vi "encoder2_test_v3.vi"() -> ()   [LabVIEW 2014]
uses:
  <vilib>/rvi/FXPMathLib/FxpSinAndCos/subVIs/nifxpmath_SinAndCos_SimConfig.ctl
  <vilib>/rvi/Emulation/niFpgaGetClockAttributes.vi
  <vilib>/rvi/Emulation/niFpgaSctlEmulationGetInTimedLoop.vi
  <vilib>/rvi/Emulation/niFpgaEmulationReportErrorSimple.vi
  <vilib>/rvi/eio/common/nirviEmuTemplateMethod_errors.vi
  <vilib>/rvi/Emulation/niFpgaProcessEmulError.vi
  <vilib>/rvi/Emulation/niFpgaCriticalErrorInLSC.vi
  <vilib>/rvi/interface/RandomDataEmulation/nirviRandomDataMultiElementFPGAFIFO.vi
  <instcachedir>/0/nirviRandomDataMultiElementFPGAFIFO_AD0CFC12EF974623A9C2E4184BC062B2.lvgen/nirviRandomDataMultiElementFPGAFIFO_AD0CFC12EF974623A9C2E4184BC062B2_028.vi
  <vilib>/rvi/interface/RandomDataEmulation/niFpgaRandomDataHandleErrors.vi
  <vilib>/rvi/FXPMathLib/FxpSinAndCos/simVIs/DllFxpSinAndCosTemp_sub.vi
  <vilib>/eio/EIONode/EIONode.xnode
  <vilib>/rvi/FXPMathLib/FxpMul/XNode/nifxpmath_Multiplier.xnode
  <vilib>/rvi/DataTransferAndStorage/Container/XNode/niFpgaContainer.xnode
  <vilib>/rvi/interface/RandomDataEmulation/nirviRandomDataFpgaMultiElementTemplate.vi
  <vilib>/rvi/FXPMathLib/FxpSinAndCos/XNode/nifxpmath_SinAndCos.xnode
  <vilib>/rvi/FXPMathLib/FxpSub/XNode/nifxpmath_Sub.xnode
  <vilib>/rvi/FXPMathLib/sim/FxpSim.dll
panel:
  in  "Tc_Mavg_mot (uSec)":i32 caption="D_d_M_avg_Tc (uSec)"
  out "omega_mot (M_avg)":fxp<+/-,40,19>
  out "D_d_mot (M_avg)":fxp<+/-,40,19>
  out "omega_mag 2":fxp<+/-,36,13>
  out "D_d_mag 2":fxp<+/-,36,16>
  in  "Tc_Mavg_mag  (uSec)":i32 caption="D_d_M_avg_Tc (uSec)"
  out "D_d_mag (M_avg)":fxp<+/-,40,19>
  out "omega_mag (M_avg)":fxp<+/-,40,19>
  in  "Velocity Est. (mag)":i16(ring) items=["T method", "Mavg method"]
  out "rad (NrTheta)":fxp<+/-,40,20>
  out "D (mm)":fxp<+/-,32,7>
  out "Dr_ramp2":fxp<+/-,64,21>
  out "Ts (s)":fxp<+/-,32,6>
  in  "Dr_ramp (mm)":fxp<+/-,33,7>
  out "Dr_ramp":fxp<+/-,64,21>
  in  "Vr (mm/s)":fxp<+/-,33,7>
  out "omega (rad/s)":fxp<+/-,36,13>
  in  "Encoder":i16(ring) items=["Motor", "Magnetic"]
  in  "Dr_step":fxp<+/-,33,7>
  out "Dr":fxp<+/-,33,10>
  in  "Command type":i16(ring) items=["Step", "Sine", "Ramp", "Ramp2"]
  out "Fmr_P":fxp<+/-,30,15>
  in  "Kp":fxp<+/-,27,14>
  out "D_error":fxp<+/-,36,11>
  out "Dr_sin_d":fxp<+/-,51,12>
  out "Sin omega":fxp<+,20,4>
  out "Dr_sin":fxp<+/-,33,10>
  in  "Sin Mag.":fxp<+/-,32,7>
  in  "Sine frequency (Hz)":fxp<+,16,5>=2.0
  out "Time now (s)":fxp<+,52,14>
  out "va":fxp<+/-,36,7>
  out "vb":fxp<+/-,37,8>
  out "vd_F":fxp<+/-,20,5>
  out "vq_F":fxp<+/-,20,5> format="%.57g"
  in  "Stop Motor":bool
  in  "Ini coe.":bool
  out "D_d_mag":fxp<+/-,36,13>
  out "omega_mag":fxp<+/-,36,13>
  out "D_mag":fxp<+/-,32,7>
  in  "Mag. factor":fxp<+/-,20,2>
  out "mt_mag.":u32
  out "D_d_mot":fxp<+/-,36,13>
  in  "Belt_screw":fxp<+/-,7,7>
  in  "Belt_motor":fxp<+/-,6,6>
  out "D_mot":fxp<+/-,32,7>
  out "rad_mag.":fxp<+/-,40,20>
  out "rad_mot":fxp<+/-,40,20>
  out "mt":u32
  out "omega_mot":fxp<+/-,36,13>
  in  "mt0":u32
  out "Mag. Encoder Position":i32
  in  "Encoder Reset":bool
  out "Encoder Position":i32
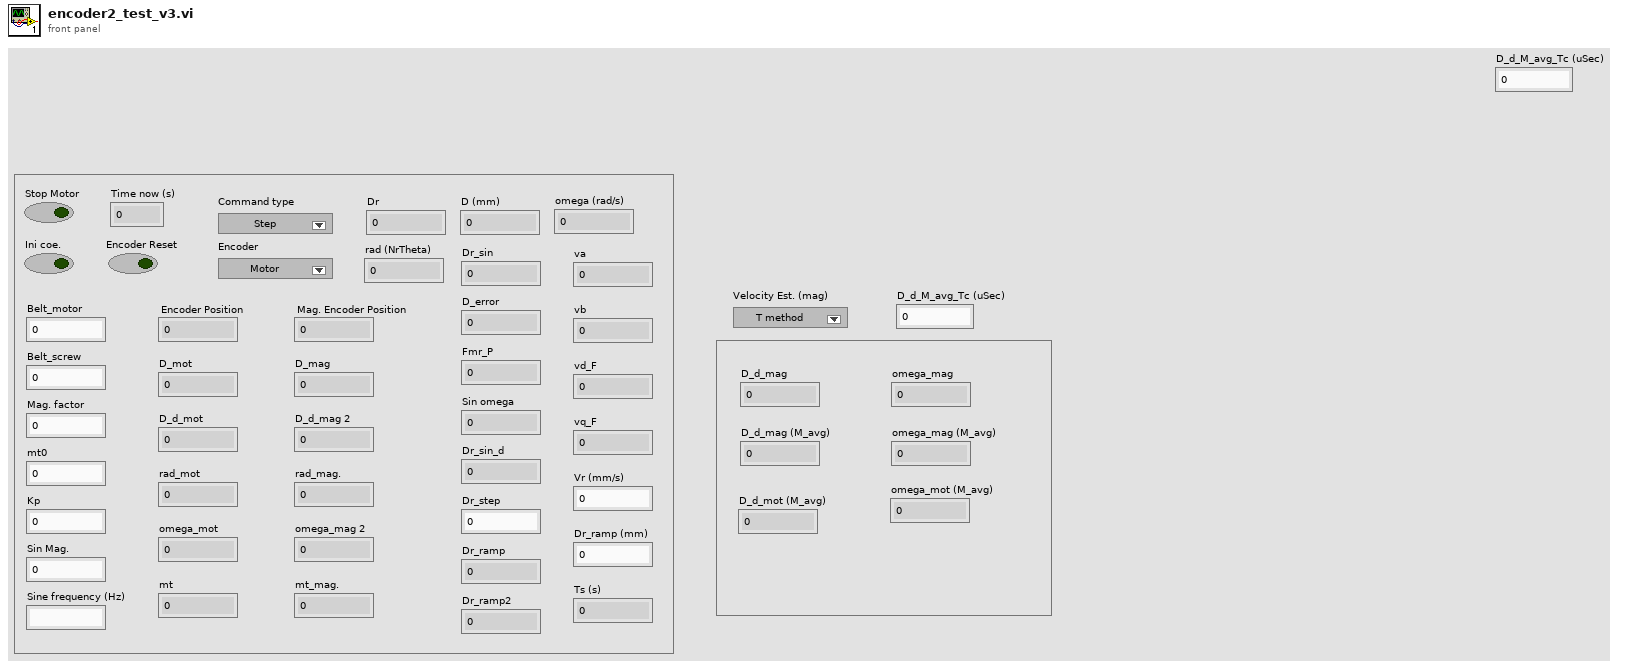
[diagram p1: front panel]
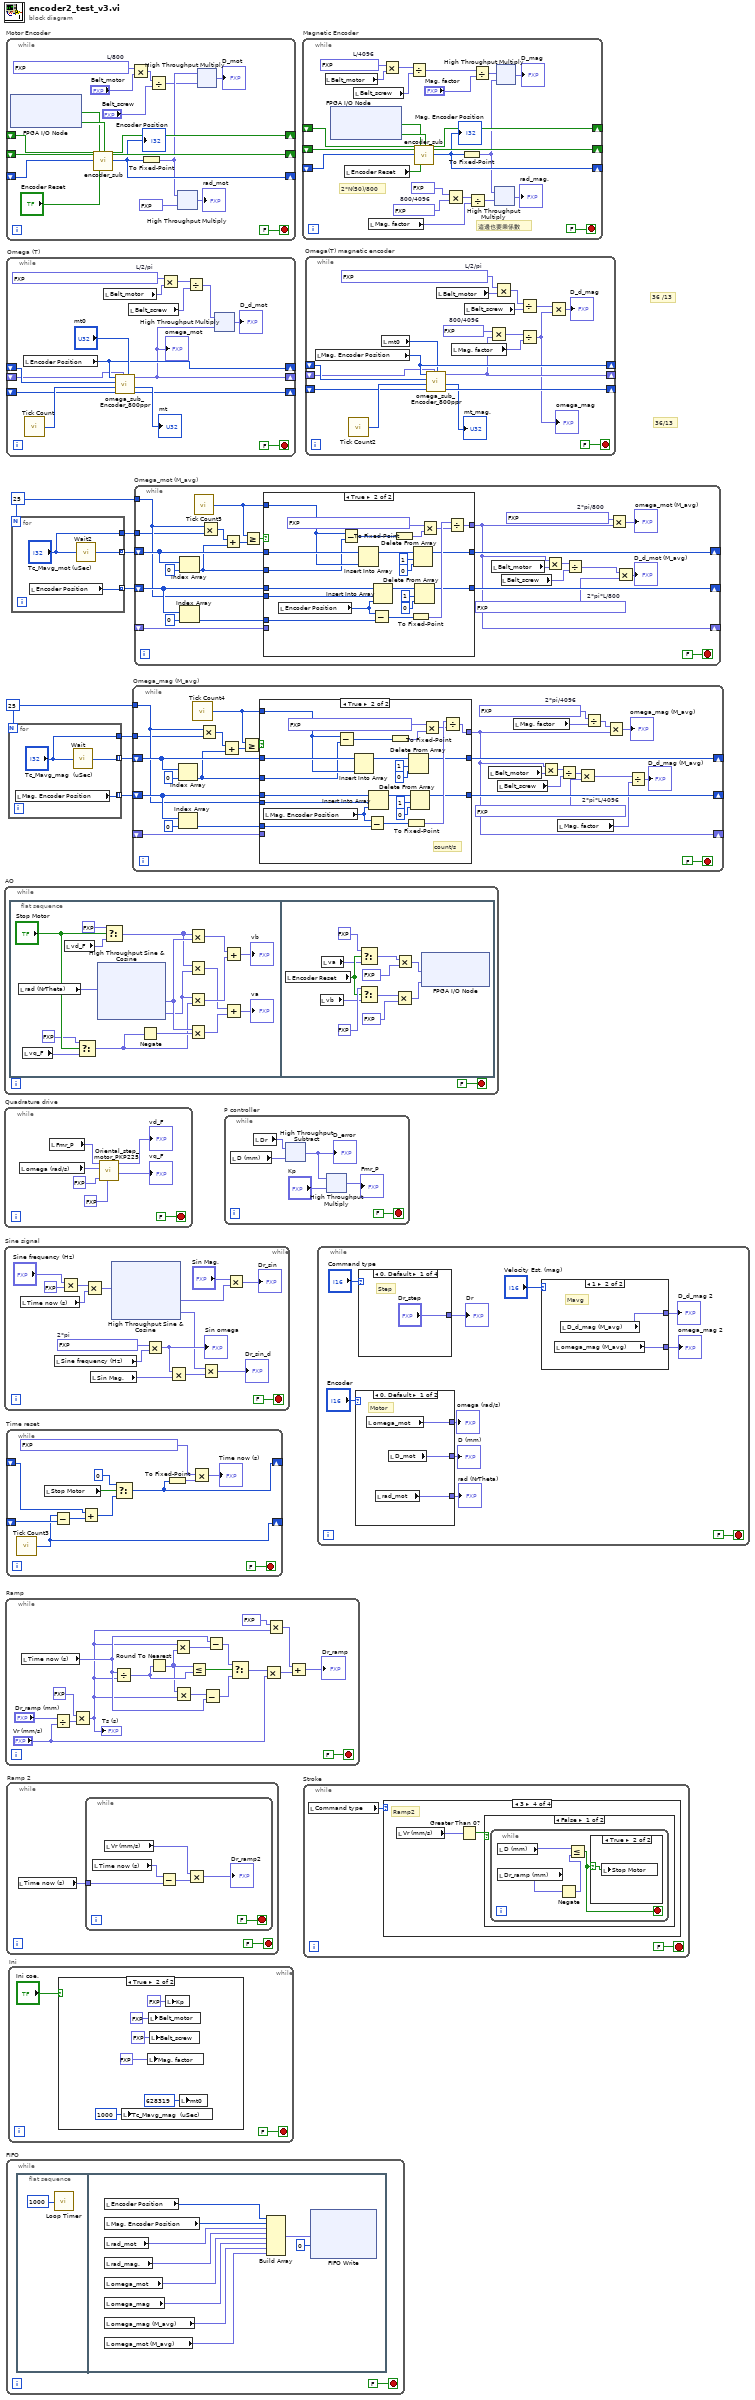
[diagram p0: block diagram]
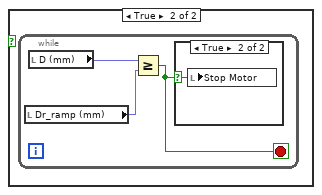
[diagram p8: hidden frame]
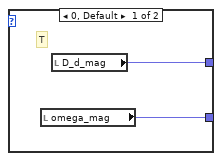
[diagram p10: hidden frame]
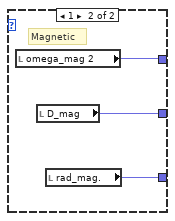
[diagram p11: hidden frame]
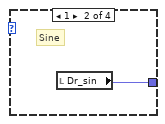
[diagram p12: hidden frame]
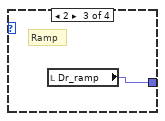
[diagram p13: hidden frame]
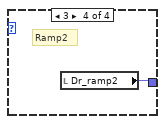
[diagram p14: hidden frame]
diagram:
  w4 = 25
  w8 = 25
  # "36/13"
  # "36 /13"
  n1 = while "AO" {
    stop <- FALSE stop-if-true
    n2 = flat-sequence {
      frame #0 {
        n3 = local read "rad (NrTheta)"() -> (w26:fxp<+/-,40,20>)
        n4 = local read "vq_F"() -> (w22:fxp<+/-,20,5>)
        n5 = local read "vd_F"() -> (w21:fxp<+/-,20,5>)
        n6 = Select(t=fxp<+,1,1> 0.0, s="Stop Motor", f=w22) -> (s? t:f=w12:fxp<+/-,20,5>)
        n7 = xnode "High Throughput Sine & Cosine"("x (pi)"=w26) -> ("sin(x)"=w16:fxp<+/-,16,2>, "cos(x)"=w14:fxp<+/-,16,2>)
        n8 = Select(t=fxp<+,1,1> 0.0, s="Stop Motor", f=w21) -> (s? t:f=w15:fxp<+/-,20,5>)
        n9 = Negate(x=w12) -> (-x=w13:fxp<+/-,21,6>)
        n10 = Multiply(x=w15, y=w16) -> (x*y=w20:fxp<+/-,36,7>)
        n11 = Multiply(x=w15, y=w14) -> (x*y=w18:fxp<+/-,36,7>)
        n12 = Multiply(x=w14, y=w12) -> (x*y=w19:fxp<+/-,36,7>)
        n13 = Multiply(x=w16, y=w13) -> (x*y=w17:fxp<+/-,35,6>)
        n14 = Add(x=w20, y=w19) -> (x+y=→"vb":fxp<+/-,37,8>)
        n15 = Add(x=w18, y=w17) -> (x+y=→"va":fxp<+/-,36,7>)
      }
      frame #1 {
        n16 = local read "Encoder Reset"() -> (w61:bool)
        n17 = local read "vb"() -> (w60:fxp<+/-,37,8>)
        n18 = local read "va"() -> (w59:fxp<+/-,36,7>)
        n19 = Select(t=fxp<+/-,20,5> 3.0 ("y"), s=w61, f=w59) -> (s? t:f=w64:fxp<+/-,36,7>)
        n20 = Select(t=fxp<+/-,20,5> 0.0 ("y"), s=w61, f=w60) -> (s? t:f=w65:fxp<+/-,37,8>)
        n21 = Multiply(x=w65, y=fxp<+/-,20,5> -0.5) -> (x*y=w57:fxp<+/-,55,11>)
        n22 = Multiply(x=w64, y=fxp<+/-,20,5> -0.5) -> (x*y=w58:fxp<+/-,55,11>)
        n23 = xnode "FPGA I/O Node"("Mod8/AO0"=w58, "Mod8/AO1"=w57) -> ()  [unwired: 2 in, 2 out]
      }
    }
  }
  n24 = while "Quadrature drive" {
    stop <- FALSE stop-if-true
    n25 = local read "omega (rad/s)"() -> (w68:fxp<+/-,36,13>)
    n26 = local read "Fmr_P"() -> (w70:fxp<+/-,30,15>)
    n27 = call "Oriental_step_motor_PKP225.vi"("F_Threshold"=fxp<+,12,12> 10.0, "dFmr"=fxp<+,1,1> 0.0 ("t"), "omega"=w68, "Fmr"=w70) -> ("vq_F"=→"vq_F":fxp<+/-,20,5>, "vd_F"=→"vd_F":fxp<+/-,20,5>)  [unwired: 6 in]
  }
  n28 = while "Sine signal" {
    stop <- FALSE stop-if-true
    w84 = fxp<+,20,3> 6.2831878662109375  # 2*pi
    n29 = local read "Time now (s)"() -> (w89:fxp<+,52,14>)
    n30 = local read "Sine frequency (Hz)"() -> (w83:fxp<+,16,5>)
    n31 = Multiply(x="Sine frequency (Hz)", y=fxp<+,1,2> 2.0 ("x")) -> (x*y=w90:fxp<+,16,6>)
    n32 = Multiply(x=w90, y=w89) -> (x*y=w88:fxp<+,64,20>)
    n33 = local read "Sin Mag."() -> (w82:fxp<+/-,32,7>)
    n34 = xnode "High Throughput Sine & Cosine"("x (pi)"=w88) -> ("sin(x)"=w86:fxp<+/-,16,2>, "cos(x)"=w79:fxp<+/-,16,2>)
    n35 = Multiply(x=w84, y=w83) -> (x*y=w81:fxp<+,36,8>)
    "Sin omega" <- w81
    n36 = Multiply(x=w81, y=w82) -> (x*y=w80:fxp<+/-,64,15>)
    n37 = Multiply(x=w79, y=w80) -> (x*y=→"Dr_sin_d":fxp<+/-,64,17>)
    n38 = Multiply(x="Sin Mag.", y=w86) -> (x*y=→"Dr_sin":fxp<+/-,48,9>)
  }
  n39 = while "Ramp" {
    stop <- FALSE stop-if-true
    n40 = local read "Time now (s)"() -> (w134:fxp<+,52,14>)
    n41 = Divide(x="Dr_ramp (mm)", y="Vr (mm/s)") -> (x/y=w123:fxp<+/-,64,34>)
    n42 = Multiply(x=fxp<+/-,3,3> 2.0, y=w123) -> (x*y=w121:fxp<+/-,64,37>)
    "Ts (s)" <- w121
    n43 = Divide(x=w134, y=w121) -> (x/y=w138:fxp<+/-,64,42>)
    n44 = Round To Nearest(number=w138) -> (nearest integer value=w137:fxp<+/-,43,43>)
    n45 = Multiply(x=w121, y=w137) -> (x*y=w136:fxp<+/-,64,79>)
    n46 = Multiply(x=w137, y=w121) -> (x*y=w135:fxp<+/-,64,79>)
    n47 = Less Or Equal?(x=w137, y=w138) -> (x <= y?=w133:bool)
    n48 = Subtract(x=w135, y=w134) -> (x-y=w131:fxp<+/-,64,80>)
    n49 = Subtract(x=w134, y=w136) -> (x-y=w132:fxp<+/-,64,80>)
    n50 = Select(t=w132, s=w133, f=w131) -> (s? t:f=w130:fxp<+/-,64,80>)
    n51 = Multiply(x=w130, y="Vr (mm/s)") -> (x*y=w127:fxp<+/-,64,87>)
    n52 = Multiply(x=fxp<+/-,2,1> -0.5, y=w121) -> (x*y=w126:fxp<+/-,64,38>)
    n53 = Add(x=w126, y=w127) -> (x+y=→"Dr_ramp":fxp<+/-,64,88>)
  }
  n54 = while "Motor Encoder" {
    shift-right: [w155] -> _
    shift-left: _ -> [w156]
    shift-right: [w154] -> _
    shift-left: _ -> [w157]
    shift-right: [w153] -> _
    shift-left: _ -> [w158]
    stop <- FALSE stop-if-true
    w144 = fxp<+/-,20,-5> 0.002499997615814209  # L/800
    n55 = xnode "FPGA I/O Node"() -> ("Mod7/DIO0"=w140:bool, "Mod7/DIO1"=w141:bool)  [unwired: 2 in, 2 out]
    n56 = call "encoder_sub.vi"("A_pre"=w156, "B_pre"=w157, "Encoder Position_pre"=w158, "A input"=w140, "Encoder Position Reset"="Encoder Reset", "B input"=w141) -> ("A"=w155:bool, "B"=w154:bool, "Encoder Position (Counts)"=w153:i32)  [unwired: 19 in]
    "Encoder Position" <- w153
    n57 = Multiply(x=w144, y="Belt_motor") -> (x*y=w146:fxp<+/-,26,1>)
    n58 = To Fixed-Point(number=w153) -> (fixed-point=w148:fxp<+/-,32,32>)  [unwired: 1 in]
    n59 = Divide(x=w146, y="Belt_screw") -> (x/y=w145:fxp<+/-,33,1>)
    n60 = xnode ("High Throughput Multiply")("x"=w148, "y"=fxp<+/-,16,1> 0.125) -> ("x*y"=→"rad_mot":fxp<+/-,48,33>)
    n61 = xnode ("High Throughput Multiply")("x"=w148, "y"=w145) -> ("x*y"=→"D_mot":fxp<+/-,64,33>)
  }
  n62 = while "Time reset" {
    shift-right: [w162] -> _
    shift-left: _ -> [w167]
    shift-right: [w165] -> _
    shift-left: _ -> [w166]
    stop <- FALSE stop-if-true
    n63 = call "Tick Count3"() -> ("Tick Count(uSec)"=w165:u32)
    n64 = local read "Stop Motor"() -> (w170:bool)
    n65 = Subtract(x=w165, y=w166) -> (x-y=w169:u32)
    n66 = Add(x=w167, y=w169) -> (x+y=w168:u32)
    n67 = Select(t=u32 0, s=w170, f=w168) -> (s? t:f=w162:u32)
    n68 = To Fixed-Point(number=w162) -> (fixed-point=w164:fxp<+,32,32>)  [unwired: 1 in]
    n69 = Multiply(x=fxp<+,20,-18> 1.0000003385357559e-06, y=w164) -> (x*y=→"Time now (s)":fxp<+,52,14>)
  }
  n70 = while "FIFO" {
    stop <- FALSE stop-if-true
    n71 = flat-sequence {
      frame #0 {
        n72 = call "Loop Timer"("Count(uSec)"=u32 1000) -> ()  [unwired: 1 out]
      }
      frame #1 {
        n73 = local read "Encoder Position"() -> (w182:i32)
        n74 = local read "Mag. Encoder Position"() -> (w181:i32)
        n75 = local read "rad_mot"() -> (w180:fxp<+/-,40,20>)
        n76 = local read "rad_mag."() -> (w179:fxp<+/-,40,20>)
        n77 = local read "omega_mot"() -> (w178:fxp<+/-,36,13>)
        n78 = local read "omega_mag"() -> (w177:fxp<+/-,36,13>)
        n79 = local read "omega_mag (M_avg)"() -> (w176:fxp<+/-,40,19>)
        n80 = local read "omega_mot (M_avg)"() -> (w173:fxp<+/-,40,19>)
        n81 = Build Array(w182, w181, w180, w179, w178, w177, w176, w173) -> (w174:fxp<+/-,55,32>[])
        n82 = xnode ("FIFO Write")("Element"=w174, "Timeout"=0) -> ()  [unwired: 1 in, 2 out]
      }
    }
  }
  n83 = while "Omega (T)" {
    shift-right: [w196] -> _
    shift-left: _ -> [w197]
    shift-right: [w185] -> _
    shift-left: _ -> [w193]
    shift-right: [w194] -> _
    shift-left: _ -> [w191]
    stop <- FALSE stop-if-true
    w190 = fxp<+/-,32,0> 0.3183098859153688  # L/2/pi
    n84 = local read "Encoder Position"() -> (w196:i32)
    n85 = call "Tick Count"() -> ("Tick Count(Ticks)"=w192:u32)
    n86 = local read "Belt_motor"() -> (w189:fxp<+/-,6,6>)
    n87 = call "omega_sub_Encoder_800ppr.vi"("mt0"="mt0", "omega_pre"=w193, "ticks_m_pre"=w191, "ticks"=w192, "count_pre"=w197, "count"=w196) -> ("ticks_m"=w194:u32, "mt"=→"mt":u32, "omega"=w185:fxp<+/-,36,13>)  [unwired: 3 in]
    "omega_mot" <- w185
    n88 = local read "Belt_screw"() -> (w187:fxp<+/-,7,7>)
    n89 = Multiply(x=w190, y=w189) -> (x*y=w188:fxp<+/-,38,6>)
    n90 = Divide(x=w188, y=w187) -> (x/y=w186:fxp<+/-,45,6>)
    n91 = xnode ("High Throughput Multiply")("x"=w186, "y"=w185) -> ("x*y"=→"D_d_mot":fxp<+/-,64,19>)
  }
  n92 = while "Ramp 2" {
    stop <- FALSE stop-if-true
    n93 = local read "Time now (s)"() -> (w200:fxp<+,52,14>)
    n94 = while {
      tunnel: w200 -> [w205]
      stop <- FALSE stop-if-true
      n95 = local read "Time now (s)"() -> (w206:fxp<+,52,14>)
      n96 = local read "Vr (mm/s)"() -> (w203:fxp<+/-,33,7>)
      n97 = Subtract(x=w206, y=w205) -> (x-y=w204:fxp<+/-,53,15>)
      n98 = Multiply(x=w203, y=w204) -> (x*y=→"Dr_ramp2":fxp<+/-,64,21>)
    }
  }
  n99 = for {
    N: w8 -> [_]
    tunnel: ["Tc_Mavg_mag  (uSec)"] -> w5
    tunnel: [w208] -> w7 mode=indexing
    tunnel: [w207] -> w6 mode=indexing
    n100 = local read "Mag. Encoder Position"() -> (w207:i32)
    n101 = call "Wait"("Count(uSec)"="Tc_Mavg_mag  (uSec)") -> ("Tick Count(uSec)"=w208:u32)
  }
  n102 = while "Ini" {
    stop <- FALSE stop-if-true
    n103 = case shown="True" "Ini coe." {
      frame False {
      }
      frame True {
        n104 = local write "Tc_Mavg_mag  (uSec)"(u32 1000 ("D_d_M_avg_Tc (uSec)")) -> ()
        n105 = local write "Mag. factor"(fxp<+/-,20,2> 1.0 ("Coorection factor")) -> ()
        n106 = local write "Belt_motor"(fxp<+/-,6,6> 14.0 ("Belt_motor")) -> ()
        n107 = local write "Belt_screw"(fxp<+/-,7,7> 36.0 ("Belt_screw")) -> ()
        n108 = local write "Kp"(fxp<+/-,27,14> 50.0 ("Kp")) -> ()
        n109 = local write "mt0"(u32 628319 ("mt0")) -> ()
      }
    }
  }
  n110 = for {
    N: w4 -> [_]
    tunnel: ["Tc_Mavg_mot (uSec)"] -> w2
    tunnel: [w219] -> w3 mode=indexing
    tunnel: [w218] -> w1 mode=indexing
    n111 = local read "Encoder Position"() -> (w218:i32)
    n112 = call "Wait2"("Count(uSec)"="Tc_Mavg_mot (uSec)") -> ("Tick Count(uSec)"=w219:u32)
  }
  n113 = while "Omega_mag (M_avg)" {
    tunnel: w8 -> [w242]
    shift-right: [w235] -> _
    shift-left: w7 -> [w246]
    shift-right: [w221] -> _
    shift-left: _ -> [w237]
    shift-right: [w236] -> _
    shift-left: w6 -> [w245]
    tunnel: w5 -> [w239]
    stop <- FALSE stop-if-true
    w226 = fxp<+/-,27,3> 0.0015339851379394531  # 2*pi/4096
    w229 = fxp<+/-,32,0> 0.003067961661145091  # 2*pi*L/4096
    n114 = Index Array(array=w246, index=0) -> (element=w240:u32)
    n115 = Index Array(array=w245, index=0) -> (element=w241:i32)
    n116 = call "Tick Count4"() -> ("Tick Count(uSec)"=w243:u32)
    n117 = Multiply(x=w242, y=w239) -> (x*y=w247:i32)
    n118 = Add(x=w247, y=w240) -> (x+y=w244:u32)
    n119 = Greater Or Equal?(x=w243, y=w244) -> (x >= y?=w238:bool)
    n120 = case shown="True" w238 {
      tunnel: w246 -> [w252 w269]
      tunnel: w245 -> [w251 w268]
      tunnel: w243 -> [_ w264]
      tunnel: w242 -> [_ w267]
      tunnel: w241 -> [_ w265]
      tunnel: w240 -> [_ w263]
      tunnel: w237 -> [w250 _]
      tunnel: [w251 w259] -> w236
      tunnel: [w252 w258] -> w235
      tunnel: [w250 w257] -> w221
      frame False {
      }
      frame True {
        # "count/s"
        n121 = local read "Mag. Encoder Position"() -> (w266:i32)
        n122 = Subtract(x=w264, y=w263) -> (x-y=w261:u32)
        n123 = Insert Into Array(array=w269, new element=w264) -> (w270:u32[])  [unwired: 1 in]
        n124 = Subtract(x=w266, y=w265) -> (x-y=w256:i32)
        n125 = Insert Into Array(array=w268, index=w267, new element=w266) -> (w271:i32[])
        n126 = To Fixed-Point(number=w261) -> (fixed-point=w253:fxp<+,32,32>)  [unwired: 1 in]
        n127 = To Fixed-Point(number=w256) -> (fixed-point=w260:fxp<+/-,32,32>)  [unwired: 1 in]
        n128 = Delete From Array(array=w270, length=1, index=0) -> (array with subset deleted=w258:u32[])  [unwired: 1 out]
        n129 = Delete From Array(array=w271, length=1, index=0) -> (array with subset deleted=w259:i32[])  [unwired: 1 out]
        n130 = Multiply(x=fxp<+/-,15,-15> 1.000240445137024e-06, y=w253) -> (x*y=w255:fxp<+/-,47,17>)
        n131 = Divide(x=w260, y=w255) -> (x/y=w257:fxp<+/-,64,32>)
      }
    }
    n132 = local read "Belt_motor"() -> (w233:fxp<+/-,6,6>)
    n133 = local read "Belt_screw"() -> (w232:fxp<+/-,7,7>)
    n134 = local read "Mag. factor"() -> (w227:fxp<+/-,20,2>)
    n135 = Multiply(x=w221, y=w233) -> (x*y=w234:fxp<+/-,64,38>)
    n136 = local read "Mag. factor"() -> (w223:fxp<+/-,20,2>)
    n137 = Divide(x=w234, y=w232) -> (x/y=w228:fxp<+/-,64,39>)
    n138 = Multiply(x=w228, y=w229) -> (x*y=w224:fxp<+/-,64,39>)
    n139 = Divide(x=w226, y=w227) -> (x/y=w225:fxp<+/-,48,22>)
    n140 = Multiply(x=w225, y=w221) -> (x*y=→"omega_mag (M_avg)":fxp<+/-,64,53>)
    n141 = Divide(x=w224, y=w223) -> (x/y=→"D_d_mag (M_avg)":fxp<+/-,64,58>)
  }
  n142 = while "Omega_mot (M_avg)" {
    tunnel: w4 -> [w292]
    shift-right: [w285] -> _
    shift-left: w3 -> [w296]
    shift-right: [w277] -> _
    shift-left: _ -> [w287]
    shift-right: [w286] -> _
    shift-left: w1 -> [w295]
    tunnel: w2 -> [w289]
    stop <- FALSE stop-if-true
    w280 = fxp<+/-,32,0> 0.015707963379099965  # 2*pi*L/800
    w278 = fxp<+/-,27,3> 0.007853984832763672  # 2*pi/800
    n143 = Index Array(array=w296, index=0) -> (element=w290:u32)
    n144 = Index Array(array=w295, index=0) -> (element=w291:i32)
    n145 = call "Tick Count5"() -> ("Tick Count(uSec)"=w293:u32)
    n146 = Multiply(x=w292, y=w289) -> (x*y=w297:i32)
    n147 = Add(x=w297, y=w290) -> (x+y=w294:u32)
    n148 = Greater Or Equal?(x=w293, y=w294) -> (x >= y?=w288:bool)
    n149 = case shown="True" w288 {
      tunnel: w296 -> [w302 w319]
      tunnel: w295 -> [w301 w318]
      tunnel: w293 -> [_ w314]
      tunnel: w292 -> [_ w317]
      tunnel: w291 -> [_ w315]
      tunnel: w290 -> [_ w313]
      tunnel: w287 -> [w300 _]
      tunnel: [w301 w309] -> w286
      tunnel: [w302 w308] -> w285
      tunnel: [w300 w307] -> w277
      frame False {
      }
      frame True {
        n150 = local read "Encoder Position"() -> (w316:i32)
        n151 = Subtract(x=w314, y=w313) -> (x-y=w311:u32)
        n152 = Insert Into Array(array=w319, new element=w314) -> (w320:u32[])  [unwired: 1 in]
        n153 = Subtract(x=w316, y=w315) -> (x-y=w306:i32)
        n154 = Insert Into Array(array=w318, index=w317, new element=w316) -> (w321:i32[])
        n155 = To Fixed-Point(number=w311) -> (fixed-point=w304:fxp<+,32,32>)  [unwired: 1 in]
        n156 = To Fixed-Point(number=w306) -> (fixed-point=w310:fxp<+/-,32,32>)  [unwired: 1 in]
        n157 = Delete From Array(array=w320, length=1, index=0) -> (array with subset deleted=w308:u32[])  [unwired: 1 out]
        n158 = Delete From Array(array=w321, length=1, index=0) -> (array with subset deleted=w309:i32[])  [unwired: 1 out]
        n159 = Multiply(x=fxp<+/-,15,-15> 1.000240445137024e-06, y=w304) -> (x*y=w305:fxp<+/-,47,17>)
        n160 = Divide(x=w310, y=w305) -> (x/y=w307:fxp<+/-,64,32>)
      }
    }
    n161 = local read "Belt_motor"() -> (w283:fxp<+/-,6,6>)
    n162 = local read "Belt_screw"() -> (w282:fxp<+/-,7,7>)
    n163 = Multiply(x=w277, y=w283) -> (x*y=w284:fxp<+/-,64,38>)
    n164 = Divide(x=w284, y=w282) -> (x/y=w276:fxp<+/-,64,39>)
    n165 = Multiply(x=w278, y=w277) -> (x*y=→"omega_mot (M_avg)":fxp<+/-,64,35>)
    n166 = Multiply(x=w276, y=w280) -> (x*y=→"D_d_mot (M_avg)":fxp<+/-,64,39>)
  }
  n167 = while "P controller" {
    stop <- FALSE stop-if-true
    n168 = local read "D (mm)"() -> (w330:fxp<+/-,32,7>)
    n169 = local read "Dr"() -> (w325:fxp<+/-,33,10>)
    n170 = xnode "High Throughput Subtract"("x"=w325, "y"=w330) -> ("x-y"=w329:fxp<+/-,36,11>)
    "D_error" <- w329
    n171 = xnode ("High Throughput Multiply")("x"=w329, "y"="Kp") -> ("x*y"=→"Fmr_P":fxp<+/-,63,25>)
  }
  n172 = while "Magnetic Encoder" {
    shift-right: [w351] -> _
    shift-left: _ -> [w352]
    shift-right: [w354] -> _
    shift-left: _ -> [w355]
    shift-right: [w350] -> _
    shift-left: _ -> [w353]
    stop <- FALSE stop-if-true
    w337 = fxp<+,20,0> 0.1953125  # 800/4096
    w347 = fxp<+/-,20,-5> 0.00048828125  # L/4096
    # "2*N(50)/800"
    # "這邊也要乘係數"
    n173 = local read "Belt_motor"() -> (w346:fxp<+/-,6,6>)
    n174 = xnode "FPGA I/O Node"() -> ("Mod7/DIO4"=w331:bool, "Mod7/DIO5"=w332:bool)  [unwired: 2 in, 2 out]
    n175 = local read "Encoder Reset"() -> (w339:bool)
    n176 = local read "Belt_screw"() -> (w344:fxp<+/-,7,7>)
    n177 = local read "Mag. factor"() -> (w333:fxp<+/-,20,2>)
    n178 = Multiply(x=w347, y=w346) -> (x*y=w345:fxp<+/-,26,1>)
    n179 = Divide(x=w345, y=w344) -> (x/y=w341:fxp<+/-,33,1>)
    n180 = call "encoder_sub.vi"("A_pre"=w352, "B_pre"=w355, "Encoder Position_pre"=w353, "A input"=w331, "Encoder Position Reset"=w339, "B input"=w332) -> ("A"=w351:bool, "B"=w354:bool, "Encoder Position (Counts)"=w350:i32)  [unwired: 19 in]
    "Mag. Encoder Position" <- w350
    n181 = Multiply(x=fxp<+/-,16,1> 0.125 ("y"), y=w337) -> (x*y=w334:fxp<+/-,36,1>)
    n182 = To Fixed-Point(number=w350) -> (fixed-point=w343:fxp<+/-,32,32>)  [unwired: 1 in]
    n183 = Divide(x=w334, y=w333) -> (x/y=w336:fxp<+/-,56,19>)
    n184 = Divide(x=w341, y="Mag. factor") -> (x/y=w342:fxp<+/-,53,19>)
    n185 = xnode ("High Throughput Multiply")("x"=w343, "y"=w336) -> ("x*y"=→"rad_mag.":fxp<+/-,64,51>)
    n186 = xnode ("High Throughput Multiply")("x"=w342, "y"=w343) -> ("x*y"=→"D_mag":fxp<+/-,64,51>)
  }
  n187 = while "Stroke" {
    stop <- FALSE stop-if-true
    n188 = local read "Command type"() -> (w357:i16)
    n189 = case shown="3" w357 {
      frame 0, Default {
        # "Step"
      }
      frame 1 {
        # "Sine"
      }
      frame 2 {
        # "Ramp"
      }
      frame 3 {
        # "Ramp2"
        n190 = local read "Vr (mm/s)"() -> (w359:fxp<+/-,33,7>)
        n191 = Greater Than 0?(x=w359) -> (x > 0?=w358:bool)
        n192 = case shown="False" w358 {
          frame False {
            n193 = while {
              stop <- w362 stop-if-true
              n194 = local read "D (mm)"() -> (w363:fxp<+/-,32,7>)
              n195 = local read "Dr_ramp (mm)"() -> (w361:fxp<+/-,33,7>)
              n196 = Negate(x=w361) -> (-x=w360:fxp<+/-,34,8>)
              n197 = Less Or Equal?(x=w363, y=w360) -> (x <= y?=w362:bool)
              n198 = case shown="True" w362 {
                selector: w362 -> [_ w364]
                frame False {
                }
                frame True {
                  n199 = local write "Stop Motor"(w364) -> ()
                }
              }
            }
          }
          frame True {
            n200 = while {
              stop <- w365 stop-if-true
              n201 = local read "Dr_ramp (mm)"() -> (w366:fxp<+/-,33,7>)
              n202 = local read "D (mm)"() -> (w367:fxp<+/-,32,7>)
              n203 = Greater Or Equal?(x=w367, y=w366) -> (x >= y?=w365:bool)
              n204 = case shown="True" w365 {
                selector: w365 -> [_ w368]
                frame False {
                }
                frame True {
                  n205 = local write "Stop Motor"(w368) -> ()
                }
              }
            }
          }
        }
      }
    }
  }
  n206 = while "Omega(T) magnetic encoder" {
    shift-right: [w383] -> _
    shift-left: _ -> [w382]
    shift-right: [w375] -> _
    shift-left: _ -> [w376]
    shift-right: [w379] -> _
    shift-left: _ -> [w380]
    stop <- FALSE stop-if-true
    w374 = fxp<+,20,0> 0.1953125  # 800/4096
    w386 = fxp<+/-,32,0> 0.3183098859153688  # L/2/pi
    n207 = local read "Mag. Encoder Position"() -> (w383:i32)
    n208 = call "Tick Count2"() -> ("Tick Count(Ticks)"=w381:u32)
    n209 = local read "mt0"() -> (w377:u32)
    n210 = call "omega_sub_Encoder_800ppr.vi"("mt0"=w377, "omega_pre"=w376, "ticks_m_pre"=w380, "ticks"=w381, "count_pre"=w382, "count"=w383) -> ("ticks_m"=w379:u32, "mt"=→"mt_mag.":u32, "omega"=w375:fxp<+/-,36,13>)  [unwired: 3 in]
    n211 = local read "Belt_motor"() -> (w385:fxp<+/-,6,6>)
    n212 = local read "Mag. factor"() -> (w369:fxp<+/-,20,2>)
    n213 = local read "Belt_screw"() -> (w384:fxp<+/-,7,7>)
    n214 = Multiply(x=w374, y=w375) -> (x*y=w370:fxp<+/-,40,14>)
    n215 = Multiply(x=w386, y=w385) -> (x*y=w387:fxp<+/-,38,6>)
    n216 = Divide(x=w387, y=w384) -> (x/y=w373:fxp<+/-,32,6>)
    n217 = Divide(x=w370, y=w369) -> (x/y=w372:fxp<+/-,61,33>)
    "omega_mag" <- w372
    n218 = Multiply(x=w373, y=w372) -> (x*y=→"D_d_mag":fxp<+/-,36,11>)
  }
  n219 = while {
    stop <- FALSE stop-if-true
    n220 = case shown="0, Default" "Encoder" {
      tunnel: [w405 w408] -> w395
      tunnel: [w404 w407] -> w394
      tunnel: [w403 w406] -> w393
      frame 0, Default {
        # "Motor"
        n221 = local read "omega_mot"() -> (w405:fxp<+/-,36,13>)
        n222 = local read "rad_mot"() -> (w403:fxp<+/-,40,20>)
        n223 = local read "D_mot"() -> (w404:fxp<+/-,32,7>)
      }
      frame 1 {
        # "Magnetic"
        n224 = local read "omega_mag 2"() -> (w408:fxp<+/-,36,13>)
        n225 = local read "D_mag"() -> (w407:fxp<+/-,32,7>)
        n226 = local read "rad_mag."() -> (w406:fxp<+/-,40,20>)
      }
    }
    "omega (rad/s)" <- w395
    "D (mm)" <- w394
    "rad (NrTheta)" <- w393
    n227 = case shown="0, Default" "Command type" {
      tunnel: ["Dr_step" w410 w411 w412] -> w397
      frame 0, Default {
        # "Step"
      }
      frame 1 {
        # "Sine"
        n228 = local read "Dr_sin"() -> (w410:fxp<+/-,33,10>)
      }
      frame 2 {
        # "Ramp"
        n229 = local read "Dr_ramp"() -> (w411:fxp<+/-,64,21>)
      }
      frame 3 {
        # "Ramp2"
        n230 = local read "Dr_ramp2"() -> (w412:fxp<+/-,64,21>)
      }
    }
    "Dr" <- w397
    n231 = case shown="1" "Velocity Est. (mag)" {
      tunnel: [w400 w402] -> w391
      tunnel: [w399 w401] -> w390
      frame 0, Default {
        # "T"
        n232 = local read "omega_mag"() -> (w399:fxp<+/-,36,13>)
        n233 = local read "D_d_mag"() -> (w400:fxp<+/-,36,13>)
      }
      frame 1 {
        # "Mavg"
        n234 = local read "omega_mag (M_avg)"() -> (w401:fxp<+/-,40,19>)
        n235 = local read "D_d_mag (M_avg)"() -> (w402:fxp<+/-,40,19>)
      }
    }
    "D_d_mag 2" <- w391
    "omega_mag 2" <- w390
  }
